vi "PathDrawerMain.vi"() -> ()   [LabVIEW 2018]
uses:
  StartingPositions.ctl
  Dawgma Programming Library/Controls/PurePursuit/PathFileData.ctl
  Dawgma Programming Library/Controls/PurePursuit/RobotNeededPathData.ctl
  <vilib>/Utility/miscctls.llb/LVBoundsTypeDef.ctl
  Robot-Project/Configuration/Constants.vi
panel:
  in  "NoUpdate":bool
  out "PathsStorage":T1[](array[typedef])=[{"RobotNeeded"={"Path"=[{67.51826792963463, 204.30852503382948}, {73.33752695702532, 204.17640783242763}, {79.12917348553499, 204.07996681682357}, {84.86117778762187, 204.06061787570727}, {90.49184817844007, 204.17225057986516}, {95.96307089902717, 204.48997502749893}, {101.19090415563274, 205.12228366964248}, {106.05199464247043, 206.2286051295332}, {110.36361644562574, 208.04511161169543}, {114.37172578385798, 210.89248691926605}, {118.17642408641785, 214.43024981480622}, {121.84478802267412, 218.4296155778484}, {125.42197657870013, 222.73663853194364}, {128.93822516173634, 227.24710298781127}, {132.4139659676452, 231.88974137154145}, {135.8631515190472, 236.6147503980893}, {139.2952430485304, 241.3855785202741}, {142.71714395845063, 246.1731860201357}, {146.13394637043862, 250.9511479319172}, {149.5499982146016, 255.691538218544}, {152.9695484837296, 260.36036298292}, {156.39736200192732, 264.9119963112372}, {159.8395350266317, 269.28183564054643}, {163.30451800782737, 273.375872369032}, {166.80445999957857, 277.0554498679603}, {170.3571607758867, 280.1148018612651}, {174.375619494585, 282.81240477743506}, {178.60376106475013, 285.2362954814753}, {182.8194665712848, 287.43019005020165}, {186.79860760663416, 289.40056942324793}, {190.27875507442488, 291.11772665764545}], "MaxVel"=150.0, "MaxAccel"=150.0, "Backwards?"=FALSE, "PointSpacing"=6.0, "LookaheadDist"=17.0, "Speed/Curve"=3.0, "SlowDistanceAtEnd"=0.0, "SlowSpeed"=15.0, "MaxDeAccel"=120.0}, "Meta"={"Path (px)"=[{97, 141}, {148, 144}, {211, 52}, {237, 42}], "RobotWidth"=33.0, "RobotLength"=38.5, "CenterOfRotYOffset"=19.5, "Roundedness"=0.8606565656565657, "StartingPositionPreset"=0}}, {"RobotNeeded"={"Path"=[{190.2787550744249, 289.3640054127199}, {186.07614817450738, 287.57919089869625}, {181.86820908755072, 285.8373118881477}, {177.6495278334142, 284.18197298538007}, {173.4145301971672, 282.65810182833405}, {169.1573974755958, 281.3126168887582}, {164.8719553893157, 280.19515659378624}, {160.55162804320773, 279.35887321854767}, {156.18924929458692, 278.86118372772233}, {151.7215043530494, 278.69831072916094}, {147.16088581833355, 278.82451340599613}, {142.5184852046493, 279.1984385240035}, {137.80416923997902, 279.78253444530395}, {133.026684408538, 280.54247263413146}, {128.1938074299499, 281.44659106907693}, {123.31249013153852, 282.46541677902627}, {118.38895358430041, 283.5712393747909}, {113.42876207603946, 284.73768817973905}, {108.43690911297081, 285.9393119731235}, {103.41790833552122, 287.15118240959157}, {98.37586932960089, 288.34852240454455}, {93.31455350147951, 289.50634008197716}, {88.2374280419424, 290.5990471382706}, {83.14769824223087, 291.6000685877231}, {78.04841600580589, 292.48141333113745}, {72.94241087303324, 293.21328024126245}, {67.75863847092603, 293.8031752482747}, {62.508875732032145, 294.2709540998106}, {57.20391482225113, 294.6346232144265}, {51.8537381760808, 294.91058865388726}, {46.46761112165648, 295.11390971178844}, {41.05423730740676, 295.2585415852749}, {35.62192615420492, 295.3575457518113}, {30.178710199232736, 295.4232806840582}, {24.732447637670262, 295.4676020403721}, {19.290933694181327, 295.5020297699594}], "MaxVel"=150.0, "MaxAccel"=150.0, "Backwards?"=FALSE, "PointSpacing"=6.0, "LookaheadDist"=17.0, "Speed/Curve"=3.0, "SlowDistanceAtEnd"=0.0, "SlowSpeed"=15.0, "MaxDeAccel"=120.0}, "Meta"={"Path (px)"=[{237, 44}, {206, 81}, {109, 29}, {42, 37}], "RobotWidth"=33.0, "RobotLength"=38.5, "CenterOfRotYOffset"=19.5, "Roundedness"=0.984969696969697, "StartingPositionPreset"=5}}, {"RobotNeeded"={"Path"=[{19.290933694181327, 295.5020297699594}, {25.011667233821314, 294.91489026868226}, {30.728152935421647, 294.3187927046234}, {36.43604092115957, 293.70465192744405}, {42.13086830735973, 293.0630905886653}, {47.80799406959849, 292.38430941833684}, {53.46250090860365, 291.65795127314783}, {59.08911131525772, 290.87293617889605}, {64.68211883509487, 290.0172832098379}, {70.23531058115069, 289.07793029495843}, {75.74187095221171, 288.0405421004314}, {81.240113340072, 286.8892926245639}, {86.73044739559474, 285.64419057963534}, {92.21315611464873, 284.3238110087589}, {97.68843015555045, 282.945570006499}, {103.15628639732084, 281.5260157214416}, {108.61673913186857, 280.0810436448667}, {114.06953940795621, 278.6261833977098}, {119.51443586582734, 277.1768101798086}, {124.95103875904077, 275.74836750511986}, {130.37878330168954, 274.3566290412284}, {135.79699940606827, 273.0179377600332}, {141.20489743697576, 271.74943958637385}, {146.60151044848593, 270.5693468230359}, {151.98567835221738, 269.4972257223495}, {157.35605871901714, 268.554294192152}, {162.71111620417892, 267.7637373962993}, {168.04908490164593, 267.15105891776346}, {173.44926104591676, 266.7078757692608}, {178.90344146020777, 266.4142240130325}, {184.4042489326938, 266.2524269236513}, {189.94502441513646, 266.2068205531521}, {195.51972173993423, 266.2635104435133}, {201.1228093724054, 266.41015930580556}, {206.74918411000075, 266.63580156156564}, {212.39409764821306, 266.93067893044196}, {218.053082726153, 267.2860914724449}, {223.7219085367435, 267.6942654904647}, {229.39645149261284, 268.1482281664267}, {235.0727578167597, 268.64170885865474}, {240.74678752259888, 269.16903578690716}, {246.41454593233095, 269.72505316763784}, {252.0719290404663, 270.3050483655174}, {257.71463906353705, 270.9046734613633}, {263.3381773893753, 271.5198771712439}, {268.93777526663223, 272.1468466517242}, {274.5082847798688, 272.78194980443004}, {280.04410508863003, 273.4216757691301}, {285.5390904772261, 274.0625870838777}, {290.98651782397354, 274.7012541041101}, {296.3788903924222, 275.3342354533153}], "MaxVel"=150.0, "MaxAccel"=150.0, "Backwards?"=TRUE, "PointSpacing"=6.0, "LookaheadDist"=17.0, "Speed/Curve"=3.0, "SlowDistanceAtEnd"=0.0, "SlowSpeed"=15.0, "MaxDeAccel"=120.0}, "Meta"={"Path (px)"=[{42, 37}, {107, 37}, {207, 82}, {358, 60}], "RobotWidth"=33.0, "RobotLength"=38.5, "CenterOfRotYOffset"=19.5, "Roundedness"=0.984969696969697, "StartingPositionPreset"=5}}, {"RobotNeeded"={"Path"=[{289.3640054127199, 276.2110960757781}, {283.89161121538694, 274.4793771139589}, {278.4253826798045, 272.77216155080026}, {272.9718885381228, 271.11525639071067}, {267.53837488594183, 269.53718906953003}, {262.1330963113174, 268.07072780126833}, {256.76586008610815, 266.7546582950609}, {251.44850479944083, 265.63586389138067}, {246.19565595648336, 264.77187218407937}, {240.7902098668073, 264.1419336162714}, {235.263847051689, 263.6975006895009}, {229.64175406548966, 263.40002247726613}, {223.94395528695148, 263.21886971120756}, {218.18640094408923, 263.12967960397833}, {212.38183590533703, 263.1130434055778}, {206.5404705353557, 263.15346144005395}, {200.67051638685254, 263.23850545062453}, {194.77863542852225, 263.358147791626}, {188.87031473608533, 263.5042248554422}, {182.9501678312608, 263.67000233440274}, {177.02217622510423, 263.84981336409123}, {171.08989455882588, 264.03874902019083}, {165.1566392195953, 264.2323883424536}, {159.22567070104284, 264.4265577087373}, {153.30037428079842, 264.61710779955916}, {147.38444449974713, 264.7996940526207}, {141.482083001354, 264.9695457680757}, {135.5982225534347, 265.1212097608314}, {129.73879137869994, 265.2482550757175}, {123.91103255880886, 265.3429243489631}, {118.12389500560474, 265.39571444716546}, {112.38851615314537, 265.3948643619865}, {106.7188221519856, 265.3257224675851}, {101.13227706543704, 265.16995828232496}, {95.65082805892156, 264.90457595641436}, {90.30207106438242, 264.5006736466917}, {85.12078578729133, 263.92189279597375}, {80.15070932417247, 263.1224387890784}, {75.44704535974232, 262.0446527497671}, {70.79261313642708, 260.6288134559805}, {66.2070365142843, 258.9757963016963}, {61.713663622712566, 257.1736951999421}, {57.34082396131312, 255.3025755179722}, {53.12326418848005, 253.43875713757274}, {49.1041948579161, 251.65899864682}], "MaxVel"=150.0, "MaxAccel"=150.0, "Backwards?"=FALSE, "PointSpacing"=6.0, "LookaheadDist"=17.0, "Speed/Curve"=3.0, "SlowDistanceAtEnd"=0.0, "SlowSpeed"=15.0, "MaxDeAccel"=120.0}, "Meta"={"Path (px)"=[{350, 59}, {304, 77}, {105, 68}, {76, 87}], "RobotWidth"=33.0, "RobotLength"=38.5, "CenterOfRotYOffset"=19.5, "Roundedness"=0.9488787878787879, "StartingPositionPreset"=5}}] {"RobotNeeded"."SlowSpeed" format="%#_13g"; "RobotNeeded"."SlowDistanceAtEnd" format="%#_13g"; "RobotNeeded"."Speed/Curve" format="%#_13g"}
  in  "Tab Control":enum32{"Path", "Load/Save"}(tab)
  in  "SetStart":bool
  in  "Deaccel":dbl=120.0 format="%#_13g"
  in  "SlowSpeed":dbl=15.0 format="%#_13g"
  in  "SlowDistanceAtEnd":dbl format="%#_13g"
  in  "Speed/Curve":dbl=3.0 format="%#_13g"
  in  "DriveBackwards?":bool
  in  "Lookahead":dbl=17.0
  out "Points (in)":cluster{dbl, dbl}[](array[cluster])=[{67.51826792963463, 204.30852503382948}, {73.33752695702532, 204.17640783242763}, {79.12917348553499, 204.07996681682357}, {84.86117778762187, 204.06061787570727}, {90.49184817844007, 204.17225057986516}, {95.96307089902717, 204.48997502749893}, {101.19090415563274, 205.12228366964248}, {106.05199464247043, 206.2286051295332}, {110.36361644562574, 208.04511161169543}, {114.37172578385798, 210.89248691926605}, {118.17642408641785, 214.43024981480622}, {121.84478802267412, 218.4296155778484}, {125.42197657870013, 222.73663853194364}, {128.93822516173634, 227.24710298781127}, {132.4139659676452, 231.88974137154145}, {135.8631515190472, 236.6147503980893}, {139.2952430485304, 241.3855785202741}, {142.71714395845063, 246.1731860201357}, {146.13394637043862, 250.9511479319172}, {149.5499982146016, 255.691538218544}, {152.9695484837296, 260.36036298292}, {156.39736200192732, 264.9119963112372}, {159.8395350266317, 269.28183564054643}, {163.30451800782737, 273.375872369032}, {166.80445999957857, 277.0554498679603}, {170.3571607758867, 280.1148018612651}, {174.375619494585, 282.81240477743506}, {178.60376106475013, 285.2362954814753}, {182.8194665712848, 287.43019005020165}, {186.79860760663416, 289.40056942324793}, {190.27875507442488, 291.11772665764545}]
  in  "Points (px)":cluster{dbl, dbl}[](array[cluster])=[{97.0, 141.0}, {148.0, 144.0}, {211.0, 52.0}, {237.0, 42.0}]
  in  "Roundedness":dbl(slide)=0.6 scale=0.6..0.997
  in  "PointSpacing":dbl=6.0 min=1.0 format="%#_13g"
  in  "Flip Path":bool
  in  "MaxVel":dbl=150.0 format="%#_13g"
  in  "Accel":dbl=150.0 format="%#_13g"
  in  "StartingPosition":T3
  in  "Multiple Paths":i32(listbox)
  in  "ExportAllToRobot":bool
  in  "LocalTempPaths":i32(listbox)
  out "standard output":string
  in  "SaveToLocal":bool
  in  "LoadFromLocal":bool
  in  "ExportToRobot":bool
  in  "LoadAllFromRobot":bool
  in  "LocalPaths":i32(listbox)
  out "standard error":string="NI Linux Real-Time (run mode)\n\nLog in with your NI-Auth credentials.\n\n"
  in  "LocalFileNames":string[](array[string])=["1LL.txt", "3RR.txt"]
  out "Path Drawer":T4(plugin-control)
  # "Double Click to add or remove paths"
  # "INSTRUCTIONS"
  # "The red line is the path that the robot recieves. Everything else is to help create that path\n\nUse the multi-line tool to draw a path. Double click to stop drawing.\nHover over a node and press backspace to remove it.\nPress I to insert a new node (at the end of the path only, for now)\n\nUse the contols to input robot width, height, and center of rotation offset,\nHow far apart the points in the \"real world units\" path are,\nWhether the robot travels on the left or right of your green lines, and\nthe roundedness of the path. (Note: point spacing affects roundedness)\n\nYou can manually edit the green node's location in the path with the Points array,\nor drag the nodes on the image\n\nPress Export To File and enter the file name (no extension) to save the path to a file in the\nThisVIsDirectory\\Paths\\ folder\n\nIf you acidentally clear your path press Z quickly to get it back"
  # "Responses of CMDs run"
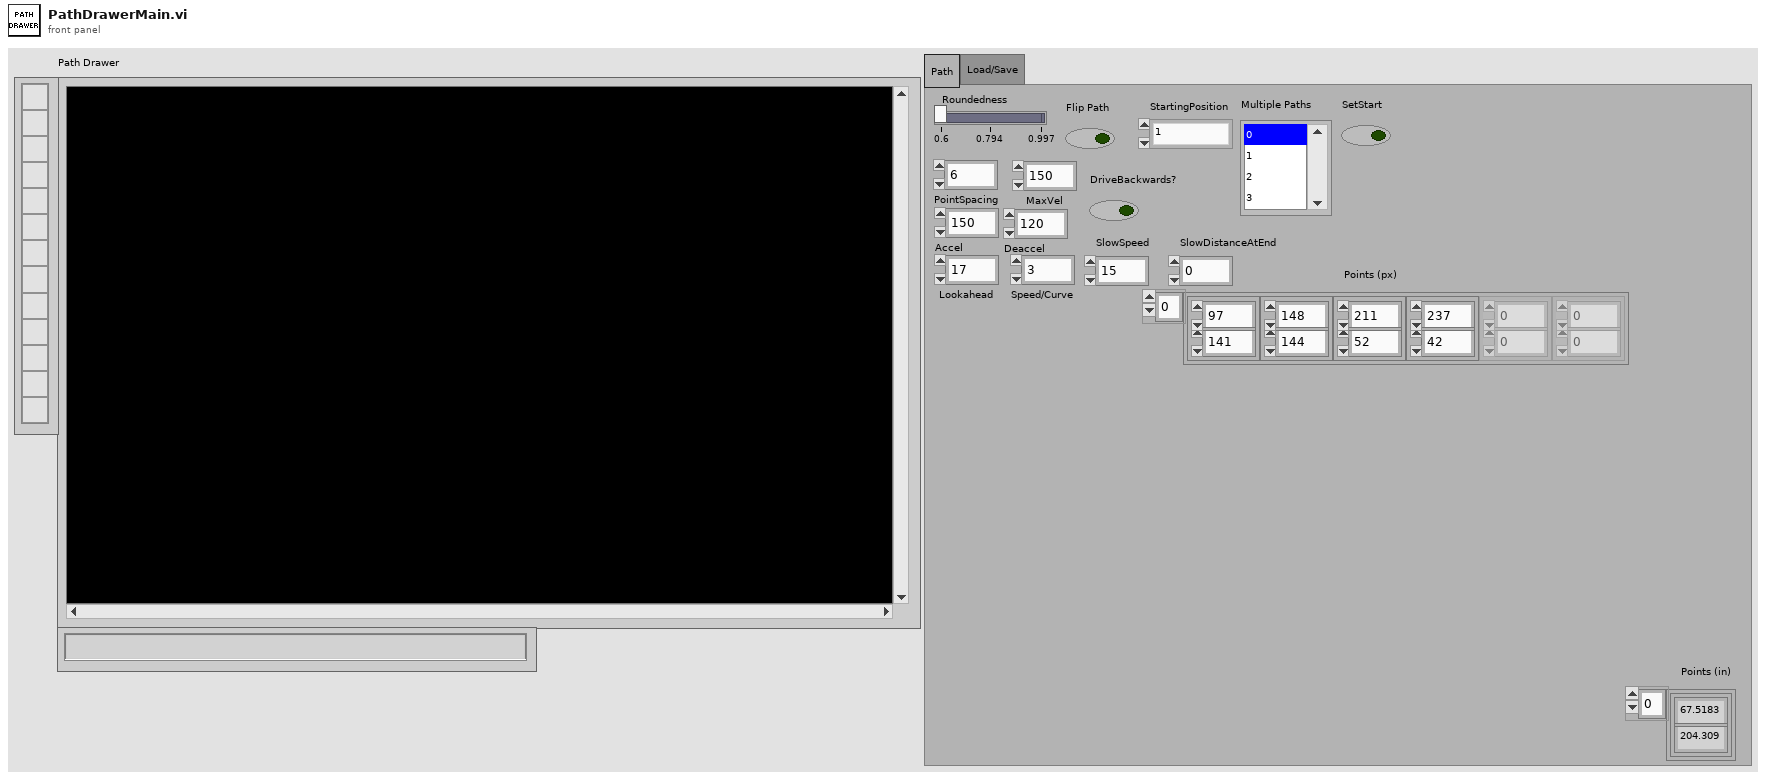
[diagram p1: front panel]
types:
  T1 = typedef "PathFileData.ctl" = cluster{"RobotNeeded":T2, "Meta":cluster{"Path (px)":cluster{i32, i32}[], "RobotWidth":dbl, "RobotLength":dbl, "CenterOfRotYOffset":dbl, "Roundedness":dbl, "StartingPositionPreset":u32}}
  T2 = typedef "RobotNeededPathData.ctl" = cluster{"Path":cluster{dbl, dbl}[], "MaxVel":dbl, "MaxAccel":dbl, "Backwards?":bool, "PointSpacing":dbl, "LookaheadDist":dbl, "Speed/Curve":dbl, "SlowDistanceAtEnd":dbl, "SlowSpeed":dbl, "MaxDeAccel":dbl}
  T3 = typedef "StartingPositions.ctl" = enum16{"1", "2", "3", "4", "5", "No Preset"}
  T4 = typedef "IMAQ Image.ctl" = refnum<image>
  T5 = typedef "Image Type" = u32
  T6 = enum16{"open", "replace", "create", "open or create", "replace or create", "replace or create with confirmation"}
  T7 = typedef "LVBoundsTypeDef.ctl" = cluster{"Width":u32, "Height":u32}
  T8 = cluster{"Global Rectangle":i32[], "Contours":cluster{"Contour Type":u32, "ROI Type":u32, "Points":i32[]}[]}
  T9 = cluster{"Contour Type":u32, "ROI Type":u32, "Points":i32[]}[]
  T10 = cluster{"Contour Type":u32, "ROI Type":u32, "Points":i32[]}
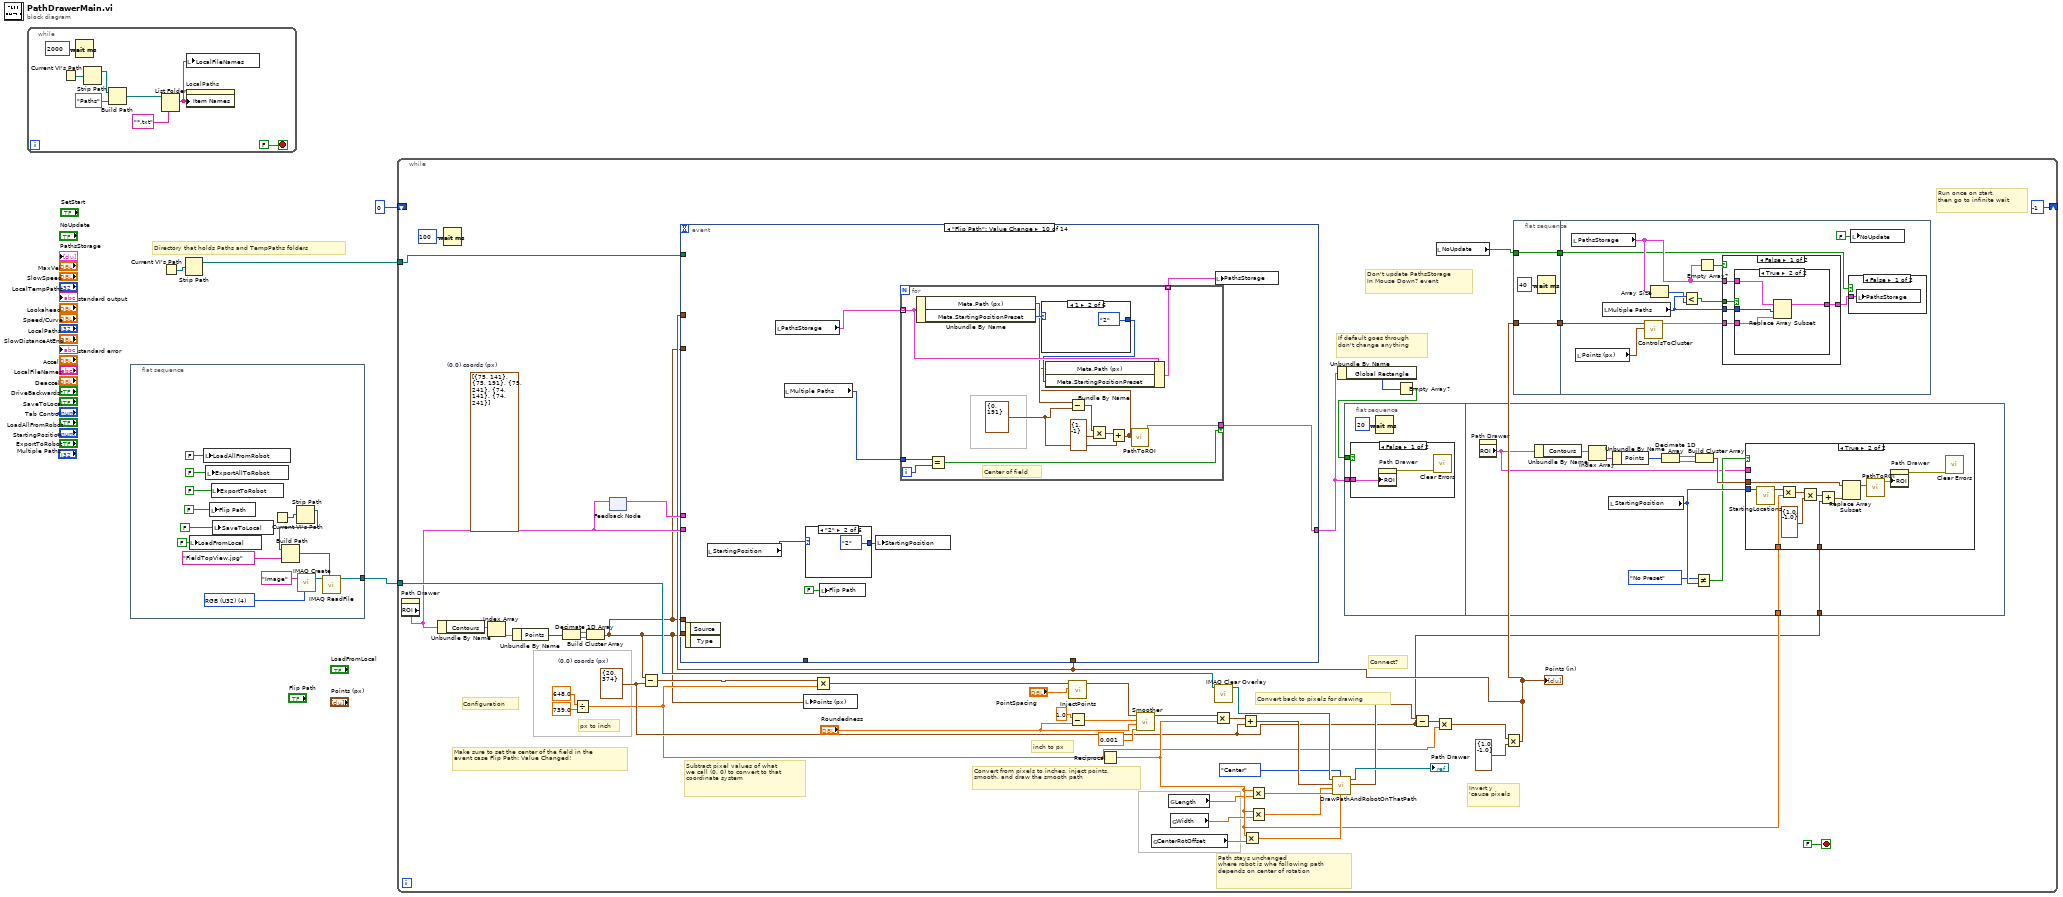
[diagram p0: block diagram]
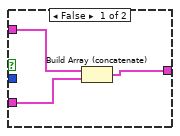
[diagram p3: hidden frame]
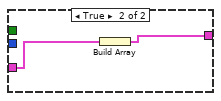
[diagram p4: hidden frame]
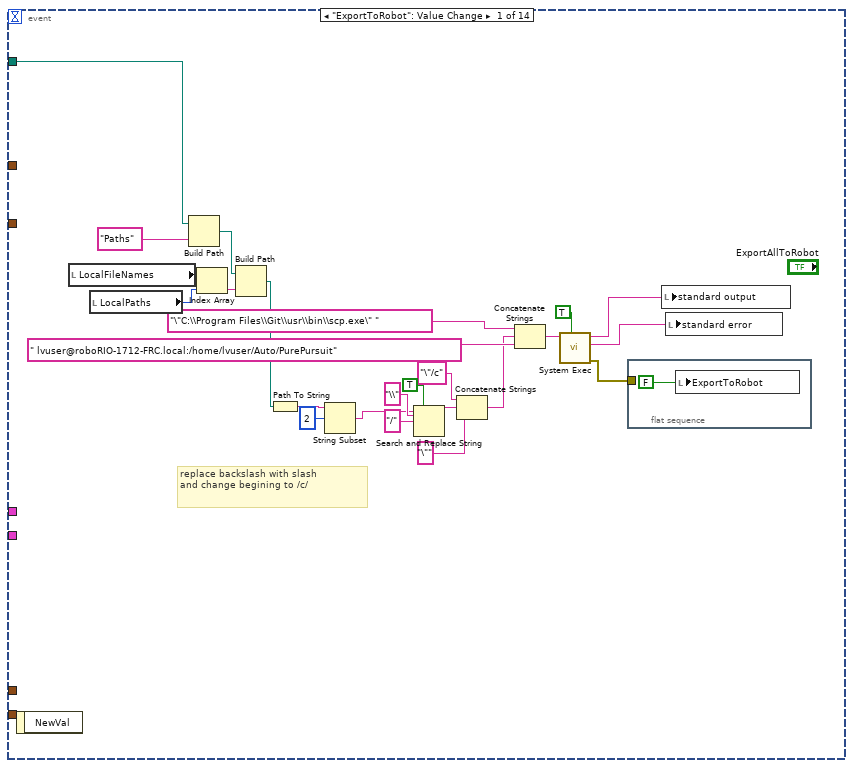
[diagram p7: hidden frame]
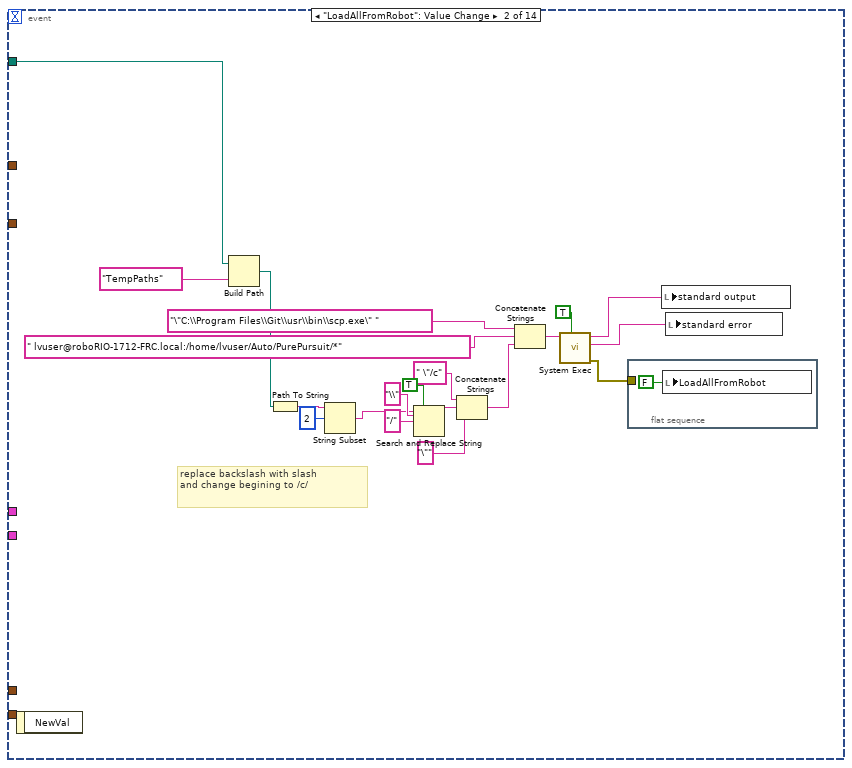
[diagram p8: hidden frame]
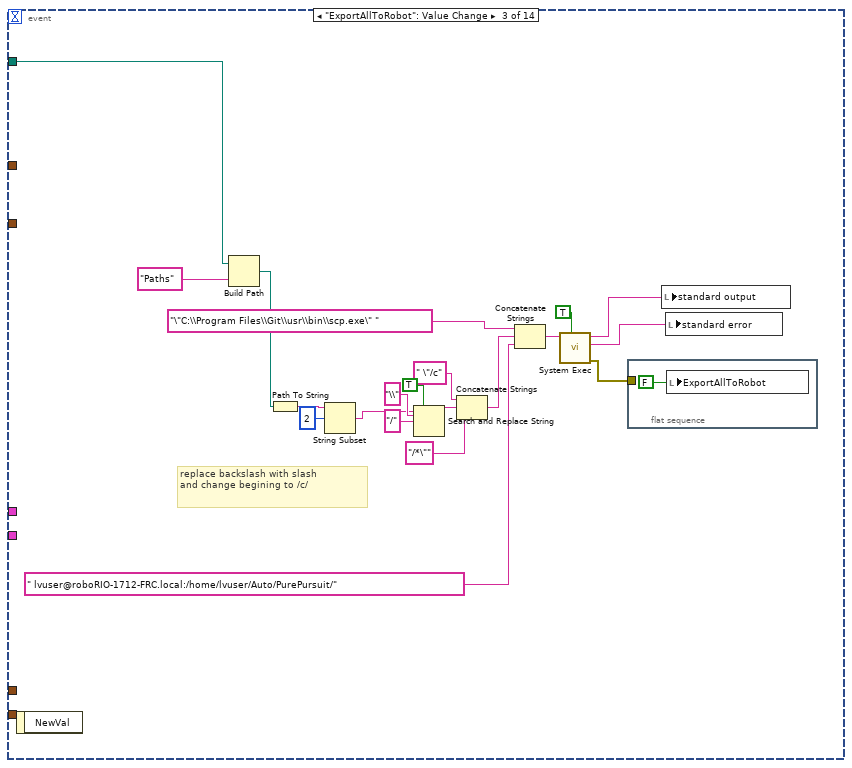
[diagram p9: hidden frame]
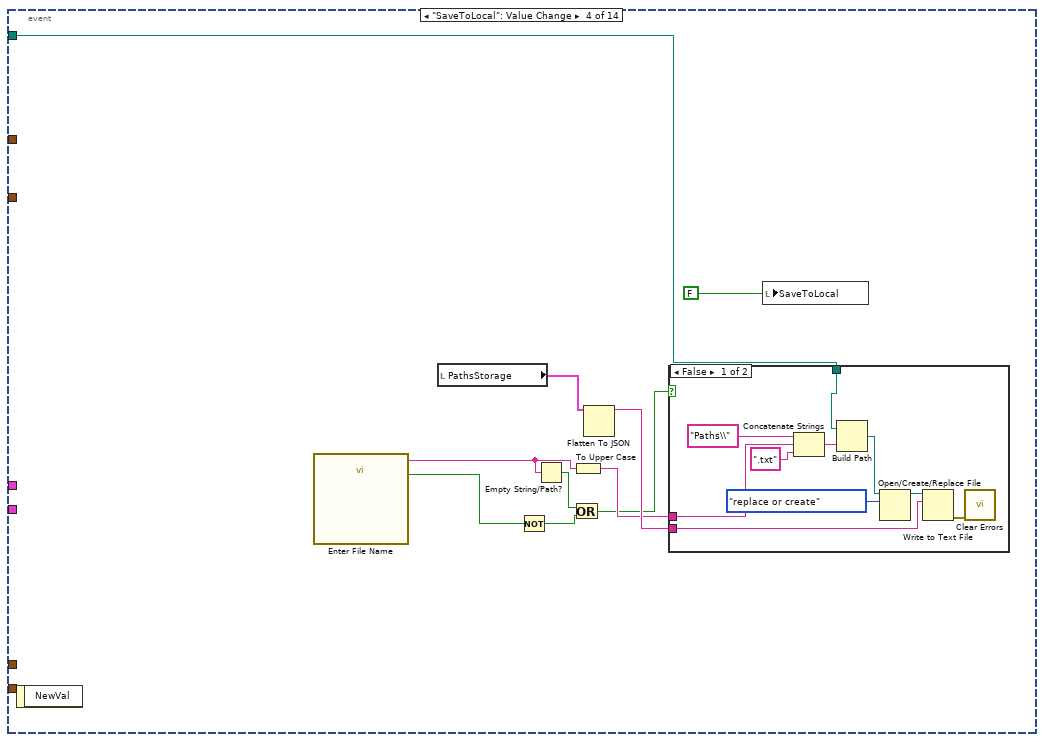
[diagram p10: hidden frame]
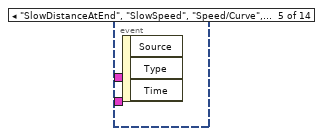
[diagram p12: hidden frame]
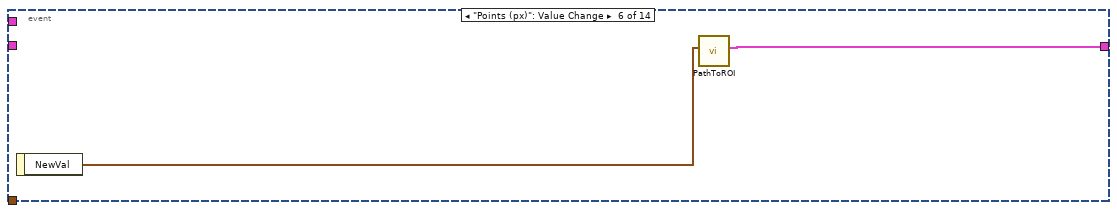
[diagram p13: hidden frame]
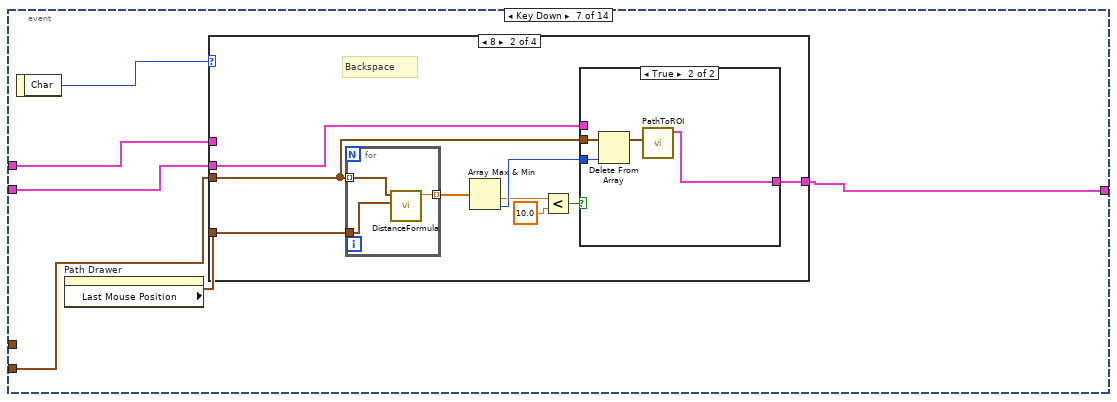
[diagram p14: hidden frame]
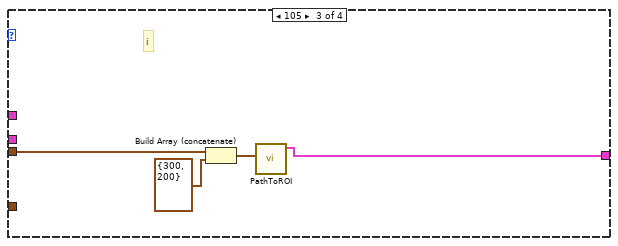
[diagram p17: hidden frame]
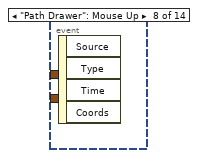
[diagram p19: hidden frame]
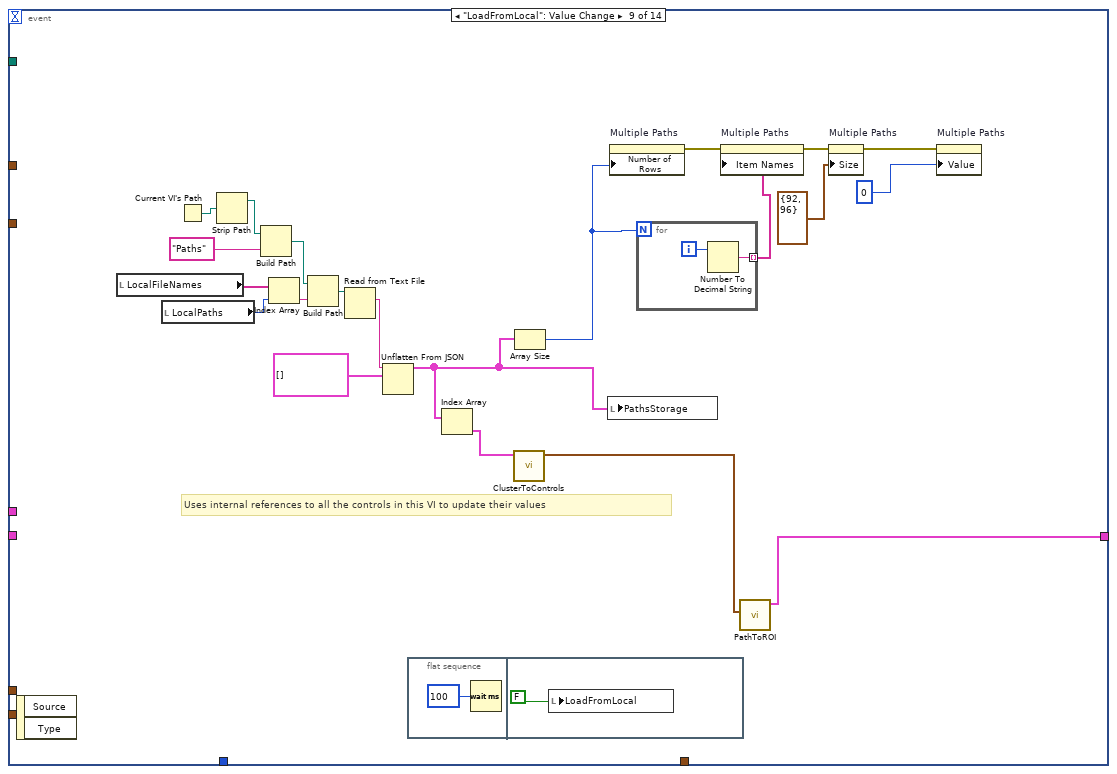
[diagram p20: hidden frame]
diagram:
  # "Directory that holds Paths and TempPaths folders"
  n1 = while {
    stop <- FALSE stop-if-true
    n2 = Current VI's Path() -> (path=w7:path)
    n3 = Wait (ms)(milliseconds to wait=u32 2000) -> ()  [unwired: 1 out]
    n4 = Strip Path(path=w7) -> (stripped path=w6:path)  [unwired: 1 out]
    n5 = Build Path(base path=w6, name or relative path="Paths") -> (appended path=w9:path)
    n6 = List Folder(path=w9, pattern="*.txt") -> (filenames=w11:string[])  [unwired: 2 in, 3 out]
    n7 = local write "LocalFileNames"(w11) -> ()
    n8 = property on="LocalPaths" class="LstBox (strict)"("Item Names"=w11) -> ()  [unwired: 2 in, 2 out]
  }
  n9 = flat-sequence {
    tunnel: [w21] -> w4
    frame #0 {
      w23 = T5 4 items=["Grayscale (U8)", "Grayscale (I16)", "Grayscale (SGL)", "Complex (CSG)", "RGB (U32)", "HSL (U32)", "RGB (U64)", "Grayscale (U16)"] ("Image Type")
      n10 = local write "LoadFromLocal"(FALSE ("Export To File")) -> ()
      n11 = local write "LoadAllFromRobot"(FALSE ("Export To File")) -> ()
      n12 = local write "ExportAllToRobot"(FALSE ("Export To File")) -> ()
      n13 = local write "Flip Path"(FALSE ("Export To File")) -> ()
      n14 = local write "ExportToRobot"(FALSE ("Export To File")) -> ()
      n15 = local write "SaveToLocal"(FALSE ("Export To File")) -> ()
      n16 = Current VI's Path() -> (path=w16:path)
      n17 = Strip Path(path=w16) -> (stripped path=w15:path)  [unwired: 1 out]
      n18 = Build Path(base path=w15, name or relative path="FieldTopView.jpg") -> (appended path=w25:path)
      n19 = call "IMAQ Create"("Image Name"="Image", "Image Type"=w23) -> ("New Image"=w22:T4)  [unwired: 3 in, 1 out]
      n20 = call "IMAQ ReadFile"("File Path"=w25, "Image"=w22) -> ("Image Out"=w21:T4)  [unwired: 5 in, 4 out]
    }
  }
  n21 = Current VI's Path() -> (path=w3:path)
  n22 = Strip Path(path=w3) -> (stripped path=w2:path)  [unwired: 1 out]
  n23 = while {
    tunnel: w4 -> [w69]
    tunnel: w2 -> [w43]
    shift-right: [-1] -> _
    shift-left: 0 -> [_]
    stop <- FALSE stop-if-true
    (unwired) cluster{i32, i32}[] [{75, 141}, {75, 191}, {75, 241}, {74, 141}, {74, 241}]  # (0,0) coords (px)
    w29 = cluster{i32, i32} {20, 374}  # (0,0) coords (px)
    # "Make sure to set the center of the field in the\nevent case Flip Path: Value Changed!"
    # "inch to px"
    # "px to inch"
    # "Configuration"
    # "Don't update PathsStorage\nIn Mouse Down? event"
    # "Run once on start,\nthen go to infinite wait"
    # "Connect?"
    # "Invert y\n'cause pixels"
    # "Path stays unchanged\nwhere robot is whe following path\ndepends on center of rotation"
    # "Convert back to pixels for drawing"
    # "If default goes through\ndon't change anything"
    # "Convert from pixels to inches, inject points,\nsmooth, and draw the smooth path"
    # "Subtract pixel values of what\nwe call (0, 0) to convert to that\ncoordinate system"
    n24 = property on="Path Drawer" class="ImageControl"() -> ("ROI"=w45:T8)  [unwired: 2 in, 2 out]
    n25 = Unbundle By Name(w45) -> ("Contours"=w75:T9)
    n26 = Wait (ms)(milliseconds to wait=u32 100) -> ()  [unwired: 1 out]
    n27 = Index Array(array=w75) -> (element=w70:T10)  [unwired: 1 in]
    n28 = Unbundle By Name(w70) -> ("Points"=w64:i32[])
    n29 = Decimate 1D Array(w64) -> (w74:i32[], w73:i32[])
    n30 = Divide(x=648.0, y=739.0) -> (x/y=w28:dbl)
    n31 = Build Cluster Array(w74, w73) -> (w27:cluster{i32, i32}[])
    n32 = feedback-in #1(w45) -> ()
    n33 = feedback #1() -> (w55:T8)  [unwired: 1 in]
    n34 = Subtract(x=w27, y=w29) -> (x-y=w65:cluster{i32, i32}[])
    n35 = local write "Points (px)"(w27) -> ()
    n36 = Multiply(x=w65, y=w28) -> (x*y=w56:cluster{dbl, dbl}[])
    n37 = call "InjectPoints.vi"("Distance"="PointSpacing", "Path"=w56) -> ("Path out"=w67:cluster{dbl, dbl}[])  [unwired: 9 in]
    n38 = Subtract(x=1.0, y="Roundedness") -> (x-y=w62:dbl)
    n39 = Reciprocal(x=w28) -> (1/x=w33:dbl)
    n40 = call "Smoother.vi"("tolerance"=0.001, "B"="Roundedness", "A"=w62, "Path"=w67) -> ("SmoothPath"=w58:cluster{dbl, dbl}[])  [unwired: 7 in]
    n41 = global read "Constants.vi" "CenterRotOffset"() -> (w30:dbl)
    n42 = global read "Constants.vi" "Length"() -> (w32:dbl)
    n43 = global read "Constants.vi" "Width"() -> (w31:dbl)
    n44 = Multiply(x=w58, y=w33) -> (x*y=w66:cluster{dbl, dbl}[])
    n45 = call "IMAQ Clear Overlay"("Image"=w69) -> ("Image Out"=w51:T4)  [unwired: 9 in, 1 out]
    n46 = Add(x=w66, y=w29) -> (x+y=w50:cluster{dbl, dbl}[])
    n47 = Multiply(x=w33, y=w30) -> (x*y=w40:dbl)
    n48 = Multiply(x=w33, y=w32) -> (x*y=w49:dbl)
    n49 = Multiply(x=w33, y=w31) -> (x*y=w41:dbl)
    n50 = call "DrawPathAndRobotOnThatPath.vi"("CenterOfRotYOffset (px)"=w40, "PathMode"=enum16{"Left", "Right", "Center"}."Center", "RobotLength (px)"=w49, "RobotWidth (px)"=w41, "Path (px)"=w50, "Image In"=w51) -> ("NewPath (px)"=w52:cluster{dbl, dbl}[], "Image Out"=→"Path Drawer":T4)  [unwired: 4 in]
    n51 = flat-sequence {
      tunnel: w44 -> [w107]
      tunnel: w42 -> [w106]
      tunnel: w33 -> [w112]
      tunnel: w29 -> [w111]
      frame #0 {
        n52 = case shown="False" w106 {
          tunnel: w107 -> [w108 _]
          frame False {
            n53 = property on="Path Drawer" class="ImageControl"("ROI"=w108) -> (error out=w109:errorcluster)  [unwired: 2 in, 1 out]
            n54 = call <vilib>:"Clear Errors.vi"("error in (no error)"=w109) -> ()  [unwired: 5 in, 2 out]
          }
          frame True {
          }
        }
        n55 = Wait (ms)(milliseconds to wait=u32 20) -> ()  [unwired: 1 out]
      }
      frame #1 {
        n56 = property on="Path Drawer" class="ImageControl"() -> ("ROI"=w113:T8)  [unwired: 2 in, 2 out]
        n57 = Unbundle By Name(w113) -> ("Contours"=w116:T9)
        n58 = Index Array(array=w116) -> (element=w119:T10)  [unwired: 1 in]
        n59 = local read "StartingPosition"() -> (w121:T3)
        n60 = Unbundle By Name(w119) -> ("Points"=w120:i32[])
        n61 = Decimate 1D Array(w120) -> (w117:i32[], w118:i32[])
        n62 = Not Equal?(x=StartingPositions."No Preset" ("StartingPosition"), y=w121) -> (x != y?=w114:bool)
        n63 = Build Cluster Array(w117, w118) -> (w115:cluster{i32, i32}[])
        n64 = case shown="True" w114 {
          tunnel: w113 -> [_ _]
          tunnel: w115 -> [_ w132]
          tunnel: w121 -> [_ w131]
          tunnel: w112 -> [_ w127]
          tunnel: w111 -> [_ w125]
          frame False {
          }
          frame True {
            n65 = call "StartingLocations.vi"("Index"=w131) -> ("Location"=w128:cluster{dbl, dbl})  [unwired: 10 in]
            n66 = Multiply(x=w128, y=w127) -> (x*y=w124:cluster{dbl, dbl})
            n67 = Multiply(x=w124, y=cluster{dbl, dbl} {1.0, -1.0}) -> (x*y=w122:cluster{dbl, dbl})
            n68 = Add(x=w122, y=w125) -> (x+y=w126:cluster{dbl, dbl})
            n69 = Replace Array Subset(array=w132, new element=w126) -> (w133:cluster{i32, i32}[])  [unwired: 1 in]
            n70 = call "PathToROI.vi"("Path In"=w133) -> ("ROI Out"=w129:T8)  [unwired: 10 in]
            n71 = property on="Path Drawer" class="ImageControl"("ROI"=w129) -> (error out=w130:errorcluster)  [unwired: 2 in, 1 out]
            n72 = call <vilib>:"Clear Errors.vi"("error in (no error)"=w130) -> ()  [unwired: 5 in, 2 out]
          }
        }
      }
    }
    n73 = Subtract(x=w52, y=w29) -> (x-y=w57:cluster{dbl, dbl}[])
    n74 = local read "NoUpdate"() -> (w34:bool)
    n75 = Multiply(x=w57, y=w28) -> (x*y=w47:cluster{dbl, dbl}[])
    n76 = Multiply(x=w47, y=cluster{dbl, dbl} {1.0, -1.0}) -> (x*y=w37:cluster{dbl, dbl}[])
    "Points (in)" <- w37
    n77 = event shown="[9] \"Flip Path\": Value Change" {
      selector: _ -> [_ _ _ _ _ _ _ _ _ _ _ _ _ _]
      dyn-events: _ -> [_ _ _ _ _ _ _ _ _ _ _ _ _ _]
      timeout: _ -> [_ _ _ _ _ _ _ _ _ _ _ _ _ _]
      tunnel: w45 -> [_ _ _ _ _ _ w228 _ _ _ _ _ w323 w363]
      tunnel: [_ _ _ _ _ w222 w225 _ w271 w279 w311 _ w322 w364] -> w44
      tunnel: w37 -> [_ _ _ _ _ _ _ _ _ _ _ _ _ _]
      tunnel: w55 -> [_ _ _ _ _ _ w224 _ _ _ _ _ _ _]
      tunnel: w27 -> [_ _ _ _ _ _ w223 _ _ _ _ _ _ _]
      tunnel: w27 -> [_ _ _ _ _ _ _ _ _ _ _ _ _ _]
      tunnel: w37 -> [_ _ _ _ _ _ _ _ _ _ _ _ _ _]
      tunnel: w43 -> [w134 w159 w180 w203 _ _ _ _ _ _ _ _ _ _]
      tunnel: [_ _ _ _ _ _ _ _ _ _ w310 _ _ _] -> _
      tunnel: w27 -> [_ _ _ _ _ _ _ _ _ _ _ _ _ _]
      event "ExportToRobot": Value Change {
        # "replace backslash with slash\nand change begining to /c/"
        n78 = event-data() -> ()  [unwired: 1 in, 1 out]
        n79 = local read "LocalFileNames"() -> (w141:string[])
        n80 = local read "LocalPaths"() -> (w142:i32)
        n81 = Build Path(base path=w134, name or relative path="Paths") -> (appended path=w144:path)
        n82 = Index Array(array=w141, index=w142) -> (element=w143:string)
        n83 = Build Path(base path=w144, name or relative path=w143) -> (appended path=w139:path)
        n84 = Path To String(path=w139) -> (string=w150:string)
        n85 = String Subset(string=w150, offset (0)=2) -> (substring=w148:string)  [unwired: 1 in]
        n86 = Search and Replace String(replace all?=TRUE ("replace all? (F)"), input string=w148, search string="\\", replace string="/" ("replace string (\"\")")) -> (result string=w147:string)  [unwired: 4 in, 3 out]
        n87 = Concatenate Strings("\"/c" ("string"), w147, "\"" ("string")) -> (w145:string)
        n88 = Concatenate Strings("\"C:\\Program Files\\Git\\usr\\bin\\scp.exe\" " ("command line"), w145, " lvuser@roboRIO-1712-FRC.local:/home/lvuser/Auto/PurePursuit" ("string")) -> (w154:string)
        n89 = call <vilib>:"System Exec.vi"("wait until completion? (T)"=TRUE, "command line"=w154) -> ("error out"=w137:errorcluster, "standard error"=w135:string, "standard output"=w136:string)  [unwired: 6 in, 1 out]
        n90 = flat-sequence {
          tunnel: w137 -> [_]
          frame #0 {
            n91 = local write "ExportToRobot"(FALSE ("Export To File")) -> ()
          }
        }
        n92 = local write "standard output"(w136) -> ()
        n93 = local write "standard error"(w135) -> ()
      }
      event "LoadAllFromRobot": Value Change {
        # "replace backslash with slash\nand change begining to /c/"
        n94 = event-data() -> ()  [unwired: 1 in, 1 out]
        n95 = Build Path(base path=w159, name or relative path="TempPaths") -> (appended path=w162:path)
        n96 = Path To String(path=w162) -> (string=w172:string)
        n97 = String Subset(string=w172, offset (0)=2) -> (substring=w170:string)  [unwired: 1 in]
        n98 = Search and Replace String(replace all?=TRUE ("replace all? (F)"), input string=w170, search string="\\", replace string="/" ("replace string (\"\")")) -> (result string=w169:string)  [unwired: 4 in, 3 out]
        n99 = Concatenate Strings(" \"/c" ("string"), w169, "\"" ("string")) -> (w160:string)
        n100 = Concatenate Strings("\"C:\\Program Files\\Git\\usr\\bin\\scp.exe\" " ("command line"), " lvuser@roboRIO-1712-FRC.local:/home/lvuser/Auto/PurePursuit/*" ("string"), w160) -> (w176:string)
        n101 = call <vilib>:"System Exec.vi"("wait until completion? (T)"=TRUE, "command line"=w176) -> ("error out"=w165:errorcluster, "standard error"=w163:string, "standard output"=w164:string)  [unwired: 6 in, 1 out]
        n102 = flat-sequence {
          tunnel: w165 -> [_]
          frame #0 {
            n103 = local write "LoadAllFromRobot"(FALSE ("Export To File")) -> ()
          }
        }
        n104 = local write "standard output"(w164) -> ()
        n105 = local write "standard error"(w163) -> ()
      }
      event "ExportAllToRobot": Value Change {
        # "replace backslash with slash\nand change begining to /c/"
        n106 = event-data() -> ()  [unwired: 1 in, 1 out]
        n107 = Build Path(base path=w180, name or relative path="Paths") -> (appended path=w183:path)
        n108 = Path To String(path=w183) -> (string=w193:string)
        n109 = String Subset(string=w193, offset (0)=2) -> (substring=w191:string)  [unwired: 1 in]
        n110 = Search and Replace String(replace all?=TRUE ("replace all? (F)"), input string=w191, search string="\\", replace string="/" ("replace string (\"\")")) -> (result string=w190:string)  [unwired: 4 in, 3 out]
        n111 = Concatenate Strings(" \"/c" ("string"), w190, "/*\"" ("string")) -> (w182:string)
        n112 = Concatenate Strings("\"C:\\Program Files\\Git\\usr\\bin\\scp.exe\" " ("command line"), w182, " lvuser@roboRIO-1712-FRC.local:/home/lvuser/Auto/PurePursuit/" ("string")) -> (w197:string)
        n113 = call <vilib>:"System Exec.vi"("wait until completion? (T)"=TRUE, "command line"=w197) -> ("error out"=w186:errorcluster, "standard error"=w184:string, "standard output"=w185:string)  [unwired: 6 in, 1 out]
        n114 = flat-sequence {
          tunnel: w186 -> [_]
          frame #0 {
            n115 = local write "ExportAllToRobot"(FALSE ("Export To File")) -> ()
          }
        }
        n116 = local write "standard output"(w185) -> ()
        n117 = local write "standard error"(w184) -> ()
      }
      event "SaveToLocal": Value Change {
        n118 = event-data() -> ()  [unwired: 1 in, 1 out]
        n119 = call "Enter File Name"() -> ("File Name"=w205:string, "Enter"=w207:bool)  [unwired: 17 in, 1 out]
        n120 = local read "PathsStorage"() -> (w201:T1[])
        n121 = Not(x=w207) -> (.not. x?=w206:bool)
        n122 = Empty String/Path?(string/path=w205) -> (empty?=w208:bool)
        n123 = Or(x=w208, y=w206) -> (x .or. y?=w202:bool)
        n124 = To Upper Case(1:w205) -> (0:w204:string)
        n125 = Flatten To JSON(anything=w201) -> (JSON string=w209:string)  [unwired: 2 in, 1 out]
        n126 = case shown="False" w202 {
          tunnel: w204 -> [w216 _]
          tunnel: w209 -> [w215 _]
          tunnel: w203 -> [w211 _]
          frame False {
            n127 = Concatenate Strings("Paths\\" ("name or relative path"), w216, ".txt" ("string")) -> (w220:string)
            n128 = Build Path(base path=w211, name or relative path=w220) -> (appended path=w214:path)
            n129 = Open/Create/Replace File(file path (use dialog)=w214, operation (0:open)=T6."replace or create") -> (refnum out=w213:refnum<file>)  [unwired: 4 in, 2 out]
            n130 = Write to Text File(file (use dialog)=w213, text=w215) -> (error out=w218:errorcluster)  [unwired: 2 in, 2 out]
            n131 = call <vilib>:"Clear Errors.vi"("error in (no error)"=w218) -> ()  [unwired: 5 in, 2 out]
          }
          frame True {
          }
        }
        n132 = local write "SaveToLocal"(FALSE ("Export To File")) -> ()
      }
      event "SlowDistanceAtEnd", "SlowSpeed", "Speed/Curve", "DriveBackwards?", "Lookahead", "Accel", "MaxVel", "Deaccel", "PointSpacing", "Roundedness": Value Change; Mouse Down; Timeout {
        n133 = event-data() -> ()  [unwired: 1 in, 3 out]
      }
      event "Points (px)": Value Change {
        n134 = event-data() -> ("NewVal"=w221:cluster{dbl, dbl}[])  [unwired: 1 in]
        n135 = call "PathToROI.vi"("Path In"=w221) -> ("ROI Out"=w222:T8)  [unwired: 10 in]
      }
      event Key Down {
        n136 = event-data() -> ("Char"=w227:i16)  [unwired: 1 in]
        n137 = property on="Path Drawer" class="ImageControl"() -> ("Last Mouse Position"=w226:cluster{"X":i32, "Y":i32})  [unwired: 2 in, 2 out]
        n138 = case shown="8" w227 {
          tunnel: w228 -> [w229 w238 _ _]
          tunnel: w223 -> [_ w237 w250 _]
          tunnel: w226 -> [_ w231 _ _]
          tunnel: [w229 w230 w247 w251] -> w225
          tunnel: w224 -> [_ _ _ w251]
          frame 0, Default {
          }
          frame 8 {
            # "Backspace"
            n139 = for {
              tunnel: w237 -> [w246] mode=indexing
              tunnel: [w245] -> w236 mode=indexing
              tunnel: w231 -> [w244]
              n140 = call "DistanceFormula.vi"("Point 2"=w244, "Point 1"=w246) -> ("Distance"=w245:dbl)  [unwired: 9 in]
            }
            n141 = Array Max & Min(array=w236) -> (min value=w234:dbl, min index (indices)=w235:i32)  [unwired: 2 out]
            n142 = Less?(x=w234, y=10.0) -> (x < y?=w232:bool)
            n143 = case shown="True" w232 {
              tunnel: w235 -> [_ w243]
              tunnel: w237 -> [_ w242]
              tunnel: w238 -> [w239 _]
              tunnel: [w239 w240] -> w230
              frame False {
              }
              frame True {
                n144 = Delete From Array(array=w242, index=w243) -> (array with subset deleted=w241:cluster{i32, i32}[])  [unwired: 1 in, 1 out]
                n145 = call "PathToROI.vi"("Path In"=w241) -> ("ROI Out"=w240:T8)  [unwired: 10 in]
              }
            }
          }
          frame 105 {
            # "i"
            n146 = Build Array (concatenate)(w250, cluster{i32, i32} {300, 200}) -> (w249:cluster{i32, i32}[])
            n147 = call "PathToROI.vi"("Path In"=w249) -> ("ROI Out"=w247:T8)  [unwired: 10 in]
          }
          frame 122 {
            # "Restore last ROI"
            # "Z"
          }
        }
      }
      event "Path Drawer": Mouse Up {
        n148 = event-data() -> ()  [unwired: 1 in, 4 out]
      }
      event "LoadFromLocal": Value Change {
        # "Uses internal references to all the controls in this VI to update their values"
        n149 = event-data() -> ()  [unwired: 1 in, 2 out]
        n150 = local read "LocalFileNames"() -> (w263:string[])
        n151 = local read "LocalPaths"() -> (w264:i32)
        n152 = Current VI's Path() -> (path=w266:path)
        n153 = Strip Path(path=w266) -> (stripped path=w265:path)  [unwired: 1 out]
        n154 = Build Path(base path=w265, name or relative path="Paths") -> (appended path=w269:path)
        n155 = Index Array(array=w263, index=w264) -> (element=w268:string)
        n156 = Build Path(base path=w269, name or relative path=w268) -> (appended path=w267:path)
        n157 = Read from Text File(file (use dialog)=w267) -> (text=w270:string)  [unwired: 3 in, 3 out]
        n158 = Unflatten From JSON(JSON string=w270, type and defaults=T1[] []) -> (value=w259:T1[])  [unwired: 5 in, 1 out]
        n159 = flat-sequence {
          frame #0 {
            n160 = Wait (ms)(milliseconds to wait=u32 100) -> ()  [unwired: 1 out]
          }
          frame #1 {
            n161 = local write "LoadFromLocal"(FALSE ("Export To File")) -> ()
          }
        }
        n162 = Index Array(array=w259) -> (element=w260:T1)  [unwired: 1 in]
        n163 = call "ClusterToControls.vi"("Path File Data"=w260) -> ("Path (px)"=w262:cluster{i32, i32}[])  [unwired: 10 in]
        n164 = Array Size(array=w259) -> (size(s)=w256:i32)
        n165 = local write "PathsStorage"(w259) -> ()
        n166 = property on="Multiple Paths" class="LstBox (strict)"("Number of Rows"=w256) -> (error out=w258:errorcluster)  [unwired: 2 in, 1 out]
        n167 = for {
          N: w256 -> [_]
          tunnel: [w273] -> w254 mode=indexing
          i -> [w274]
          n168 = Number To Decimal String(number=w274) -> (decimal integer string=w273:string)  [unwired: 1 in]
        }
        n169 = property on="Multiple Paths" class="LstBox (strict)"(error in=w258, "Item Names"=w254) -> (error out=w257:errorcluster)  [unwired: 1 in, 1 out]
        n170 = call "PathToROI.vi"("Path In"=w262) -> ("ROI Out"=w271:T8)  [unwired: 10 in]
        n171 = property on="Multiple Paths" class="LstBox (strict)"(error in=w257, "Size"=T7 {"Width"=92, "Height"=96}) -> (error out=w252:errorcluster)  [unwired: 1 in, 1 out]
        n172 = property on="Multiple Paths" class="LstBox (strict)"(error in=w252, "Value"=0 ("Active Row:Active Row Number")) -> ()  [unwired: 1 in, 2 out]
      }
      event "Flip Path": Value Change {
        n173 = event-data() -> ()  [unwired: 1 in, 2 out]
        n174 = local read "StartingPosition"() -> (w281:T3)
        n175 = local read "PathsStorage"() -> (w280:T1[])
        n176 = local read "Multiple Paths"() -> (w277:i32)
        n177 = case shown="\"2\"" w281 {
          tunnel: [StartingPositions."3" ("StartingPosition") StartingPositions."2" ("StartingPosition") StartingPositions."1" ("StartingPosition") StartingPositions."5" ("StartingPosition") StartingPositions."4" ("StartingPosition") StartingPositions."No Preset" ("StartingPosition")] -> w282
          frame "1", Default {
          }
          frame "2" {
          }
          frame "3" {
          }
          frame "4" {
          }
          frame "5" {
          }
          frame "No Preset" {
          }
        }
        n178 = local write "Flip Path"(FALSE ("Export To File")) -> ()
        n179 = local write "StartingPosition"(w282) -> ()
        n180 = for {
          tunnel: w280 -> [w296] mode=indexing
          tunnel: [w290] -> w279 if=w284
          tunnel: [w287] -> w278 mode=indexing
          tunnel: w277 -> [w285]
          i -> [w286]
          w292 = cluster{i32, i32} {0, 191}
          # "Center of field"
          n181 = Unbundle By Name(w296) -> ("Meta.Path (px)"=w289:cluster{i32, i32}[], "Meta.StartingPositionPreset"=w297:u32)
          n182 = Equal?(x=w285, y=w286) -> (x = y?=w284:bool)
          n183 = case shown="1" w297 {
            tunnel: [StartingPositions."3" ("StartingPosition") StartingPositions."2" ("StartingPosition") StartingPositions."1" ("StartingPosition") StartingPositions."5" ("StartingPosition") StartingPositions."4" ("StartingPosition") StartingPositions."No Preset" ("StartingPosition")] -> w295
            frame 0, Default {
            }
            frame 1 {
            }
            frame 2 {
            }
            frame 3 {
            }
            frame 4 {
            }
            frame 5 {
            }
          }
          n184 = Subtract(x=w289, y=w292) -> (x-y=w294:cluster{i32, i32}[])
          n185 = Multiply(x=w294, y=cluster{i32, i32} {1, -1}) -> (x*y=w293:cluster{i32, i32}[])
          n186 = Add(x=w293, y=w292) -> (x+y=w288:cluster{i32, i32}[])
          n187 = Bundle By Name(cluster=w296, "Meta.Path (px)"=w288, "Meta.StartingPositionPreset"=w295) -> (w287:T1)
          n188 = call "PathToROI.vi"("Path In"=w288) -> ("ROI Out"=w290:T8)  [unwired: 10 in]
        }
        n189 = local write "PathsStorage"(w278) -> ()
      }
      event "Multiple Paths": Value Change {
        n190 = event-data() -> ("NewVal"=w310:i32)  [unwired: 1 in, 5 out]
        n191 = local read "Multiple Paths"() -> (w312:i32)
        n192 = local read "PathsStorage"() -> (w313:T1[])
        n193 = Index Array(array=w313, index=w312) -> (element=w315:T1)
        n194 = call "ClusterToControls.vi"("Path File Data"=w315) -> ("Path (px)"=w314:cluster{i32, i32}[])  [unwired: 10 in]
        n195 = call "PathToROI.vi"("Path In"=w314) -> ("ROI Out"=w311:T8)  [unwired: 10 in]
      }
      event "Multiple Paths": Mouse Down? {
        # "2 for right click, 1 for regular click.\nBy turning double click into right click we open the options menu"
        n196 = event-data() -> ("Mods"=w321:cluster{"Double Click":bool, "Menu Key":bool})  [unwired: 1 in, 7 out]
        n197 = Unbundle By Name(w321) -> ("Double Click"=w320:bool)
        n198 = Select(t=u16 2 ("Button"), s=w320, f=u16 1) -> (s? t:f=w317:u16)
        n199 = local write "NoUpdate"(TRUE ("NoUpdate")) -> ()
        n200 = event-data("Button"=w317) -> ()  [unwired: 1 in, 1 out]
      }
      event "Multiple Paths": Shortcut Menu Selection (User) {
        n201 = event-data() -> ("ItemTag"=w326:string)  [unwired: 1 in, 7 out]
        n202 = local read "PathsStorage"() -> (w325:T1[])
        n203 = case shown="\"New Path\", Default" w326 {
          tunnel: w325 -> [w329 w360]
          tunnel: [w328 w348] -> w324
          tunnel: w323 -> [_ _]
          tunnel: [_ w347] -> w322
          frame "New Path", Default {
            n204 = Array Size(array=w329) -> (size(s)=w335:i32)
            n205 = Increment(x=w335) -> (x+1=w342:i32)
            n206 = Decrement(x=w335) -> (x-1=w334:i32)
            n207 = Index Array(array=w329, index=w334) -> (element=w338:T1)
            n208 = Unbundle By Name(w338) -> ("Meta.Path (px)"=w337:cluster{i32, i32}[])
            n209 = for {
              N: w342 -> [_]
              tunnel: [w345] -> w344 mode=indexing
              i -> [w346]
              n210 = Number To Decimal String(number=w346) -> (decimal integer string=w345:string)  [unwired: 1 in]
            }
            n211 = property on="Multiple Paths" class="LstBox (strict)"("Number of Rows"=w342) -> (error out=w341:errorcluster)  [unwired: 2 in, 1 out]
            n212 = Reverse 1D Array(array=w337) -> (reversed array=w336:cluster{i32, i32}[])
            n213 = Index Array(array=w336) -> (element=w333:cluster{i32, i32})  [unwired: 1 in]
            n214 = Add(x=w333, y=cluster{i32, i32} {-60, 0}) -> (x+y=w331:cluster{i32, i32})
            n215 = property on="Multiple Paths" class="LstBox (strict)"(error in=w341, "Item Names"=w344) -> (error out=w340:errorcluster)  [unwired: 1 in, 1 out]
            n216 = Build Array(w333, w331) -> (w330:cluster{i32, i32}[])
            n217 = Bundle By Name(cluster=w338, "Meta.StartingPositionPreset"=StartingPositions."No Preset" ("StartingPosition"), "Meta.Path (px)"=w330) -> (w339:T1)
            n218 = Build Array (concatenate)(w329, w339) -> (w328:T1[])
            n219 = property on="Multiple Paths" class="LstBox (strict)"(error in=w340, "Size"=T7 {"Width"=92, "Height"=96}) -> ()  [unwired: 1 in, 2 out]
          }
          frame "Remove Path" {
            n220 = local read "Multiple Paths"() -> (w359:i32)
            n221 = Delete From Array(array=w360, length=1, index=w359) -> (array with subset deleted=w348:T1[])  [unwired: 1 out]
            n222 = Index Array(array=w348) -> (element=w349:T1)  [unwired: 1 in]
            n223 = Array Size(array=w348) -> (size(s)=w353:i32)
            n224 = for {
              N: w353 -> [_]
              tunnel: [w361] -> w354 mode=indexing
              i -> [w362]
              n225 = Number To Decimal String(number=w362) -> (decimal integer string=w361:string)  [unwired: 1 in]
            }
            n226 = property on="Multiple Paths" class="LstBox (strict)"("Number of Rows"=w353) -> (error out=w356:errorcluster)  [unwired: 2 in, 1 out]
            n227 = call "ClusterToControls.vi"("Path File Data"=w349) -> ("Path (px)"=w350:cluster{i32, i32}[])  [unwired: 10 in]
            n228 = call "PathToROI.vi"("Path In"=w350) -> ("ROI Out"=w347:T8)  [unwired: 10 in]
            n229 = property on="Multiple Paths" class="LstBox (strict)"(error in=w356, "Item Names"=w354) -> (error out=w355:errorcluster)  [unwired: 1 in, 1 out]
            n230 = property on="Multiple Paths" class="LstBox (strict)"(error in=w355, "Size"=T7 {"Width"=92, "Height"=96}) -> (error out=w351:errorcluster)  [unwired: 1 in, 1 out]
            n231 = property on="Multiple Paths" class="LstBox (strict)"(error in=w351, "Value"=0 ("Active Row:Active Row Number")) -> ()  [unwired: 1 in, 2 out]
          }
        }
        n232 = local write "PathsStorage"(w324) -> ()
      }
      event "SetStart": Value Change {
        n233 = event-data() -> ()  [unwired: 1 in, 6 out]
        n234 = local read "Multiple Paths"() -> (w365:i32)
        n235 = Not Equal To 0?(x=w365) -> (x != 0?=w366:bool)
        n236 = case shown="True" w366 {
          tunnel: w365 -> [_ w371]
          tunnel: [_ w367] -> w364
          tunnel: w363 -> [_ _]
          frame False {
          }
          frame True {
            n237 = Decrement(x=w371) -> (x-1=w380:i32)
            n238 = local read "PathsStorage"() -> (w370:T1[])
            n239 = Index Array(array=w370, index #1=w380, index #2=w371) -> (element #1=w379:T1, element #2=w373:T1)
            n240 = Unbundle By Name(w373) -> ("Meta.Path (px)"=w376:cluster{i32, i32}[])
            n241 = Unbundle By Name(w379) -> ("Meta.Path (px)"=w378:cluster{i32, i32}[])
            n242 = Reverse 1D Array(array=w378) -> (reversed array=w377:cluster{i32, i32}[])
            n243 = Index Array(array=w377) -> (element=w375:cluster{i32, i32})  [unwired: 1 in]
            n244 = Replace Array Subset(array=w376, new element=w375, index=0) -> (w368:cluster{i32, i32}[])
            n245 = Bundle By Name(cluster=w373, "Meta.Path (px)"=w368) -> (w372:T1)
            n246 = Replace Array Subset(array=w370, new element=w372, index=w371) -> (w369:T1[])
            n247 = local write "PathsStorage"(w369) -> ()
            n248 = call "PathToROI.vi"("Path In"=w368) -> ("ROI Out"=w367:T8)  [unwired: 10 in]
          }
        }
        n249 = flat-sequence {
          frame #0 {
            n250 = Wait (ms)(milliseconds to wait=u32 100) -> ()  [unwired: 1 out]
          }
          frame #1 {
            n251 = local write "SetStart"(FALSE ("SetStart")) -> ()
          }
        }
      }
    }
    n252 = Unbundle By Name(w44) -> ("Global Rectangle"=w59:i32[])
    n253 = Empty Array?(array=w59) -> (empty?=w42:bool)
    n254 = flat-sequence {
      tunnel: w34 -> [w77]
      tunnel: w37 -> [w78]
      tunnel: [w78] -> w36
      tunnel: [w77] -> w35
      tunnel: w36 -> [w81]
      tunnel: w35 -> [w80]
      frame #0 {
        n255 = Wait (ms)(milliseconds to wait=u32 40) -> ()  [unwired: 1 out]
      }
      frame #1 {
        n256 = local read "PathsStorage"() -> (w83:T1[])
        n257 = local read "Points (px)"() -> (w89:cluster{dbl, dbl}[])
        n258 = local read "Multiple Paths"() -> (w85:i32)
        n259 = call "ControlsToCluster.vi"("Path (px)"=w89, "Path (in)"=w81) -> ("Path File Data"=w87:T1)  [unwired: 9 in]
        n260 = Array Size(array=w83) -> (size(s)=w84:i32)
        n261 = Less?(x=w85, y=w84) -> (x < y?=w88:bool)
        n262 = Empty Array?(array=w83) -> (empty?=w86:bool)
        n263 = case shown="False" w86 {
          tunnel: [w95 w103] -> w82
          tunnel: w85 -> [w94 _]
          tunnel: w88 -> [w93 _]
          tunnel: w87 -> [w92 w104]
          tunnel: w83 -> [w91 _]
          frame False {
            n264 = case shown="True" w93 {
              tunnel: w91 -> [w97 w102]
              tunnel: w92 -> [w98 w100]
              tunnel: [w96 w101] -> w95
              tunnel: w94 -> [_ w99]
              frame False {
                n265 = Build Array (concatenate)(w97, w98) -> (w96:T1[])
              }
              frame True {
                n266 = Replace Array Subset(array=w102, new element=w100, index=w99) -> (w101:T1[])
              }
            }
          }
          frame True {
            n267 = Build Array(w104) -> (w103:T1[])
          }
        }
        n268 = case shown="False" w80 {
          tunnel: w82 -> [w90 _]
          frame False {
            n269 = local write "PathsStorage"(w90) -> ()
          }
          frame True {
          }
        }
        n270 = local write "NoUpdate"(FALSE ("NoUpdate")) -> ()
      }
    }
  }
